vi "WriteFPS.vi"(7 "force?":bool, 8 "error in":errorcluster, 10 "FPS":dbl, 11 "camera.nit in":refnum<class "camera.lvclass">) -> (0 "error out":errorcluster)   [LabVIEW 2020, in "camera.lvclass"]
uses:
  camera.lvclass
  abe412ce-77be-482c-90d9-2c09ee94f937.vi
  camera.lvclass/camera.ctl
  lib/O-PL.dll
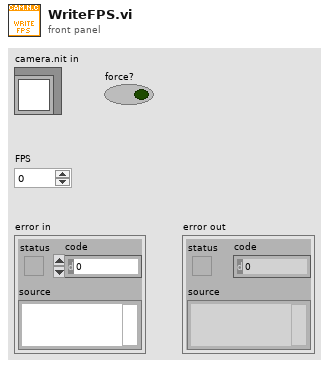
[diagram p1: front panel]
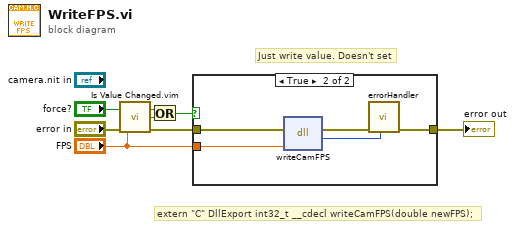
[diagram p0: block diagram]
diagram:
  # "Just write value. Doesn't set"
  # "extern \"C\" DllExport int32_t __cdecl writeCamFPS(double newFPS);"
  n1 = call "Is Value Changed.vim"("value"="FPS") -> ("changed or first call?"=w6:bool)
  n2 = Or(x="force?", y=w6) -> (x .or. y?=w2:bool)
  n3 = case shown="True" w2 {
    tunnel: "FPS" -> [_ w8]
    tunnel: "error in" -> [w7 w11]
    tunnel: [w7 w10] -> w3
    frame False {
    }
    frame True {
      n4 = dll-call lib="D:/UNSW - New/v0.8.3/lib/O-PL.dll" fn="writeCamFPS"(error in=w11, "FPS"=w8) -> (error out=w10:errorcluster, "return type"=w9:i32)  [unwired: 3 in, 1 out]
      n5 = call "errorHandler.vi"("code"=w9) -> ()  [unwired: 10 in, 1 out]
    }
  }
  "error out" <- w3
